vi "Smooth Ramp by Samples.vi"(8 "error in (no error)":errorcluster, 9 "End":dbl[](array[numeric]), 10 "Start":dbl[](array[numeric]), 11 "Generator in":refnum<class "Generator.lvclass">) -> (0 "Error out":errorcluster, 2 "Waveforms out":waveform(dbl)[](array[waveform]), 3 "Generator out":refnum<class "Generator.lvclass">)   [LabVIEW 2019, in "Generator.lvclass"]
uses:
  Generator.lvclass
  Generator.lvclass/Generator.ctl
  <vilib>/Analysis/NI_AALBase.lvlib
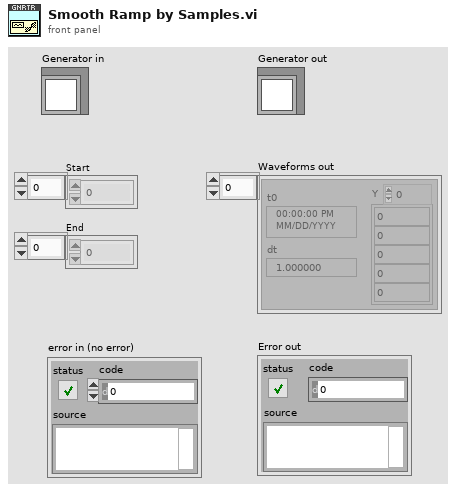
[diagram p1: front panel]
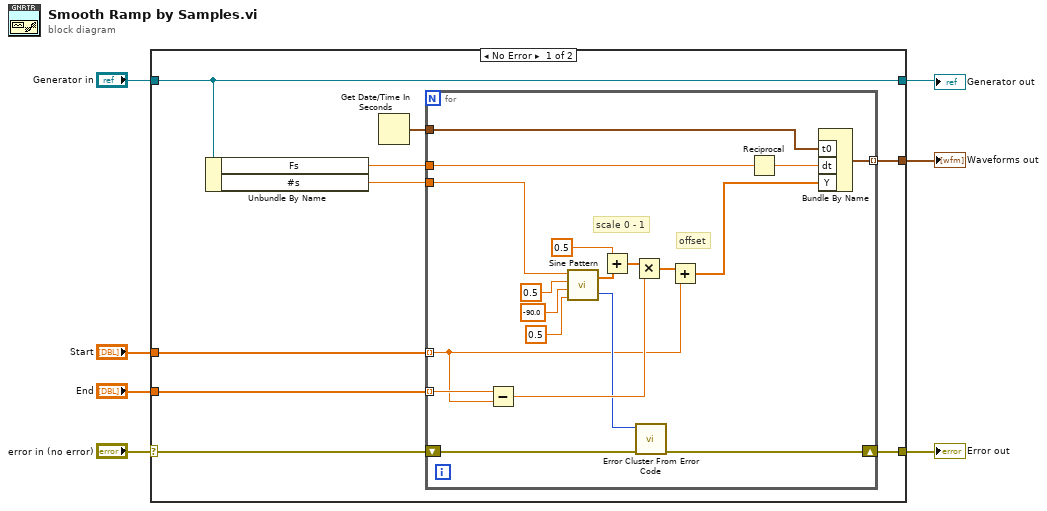
[diagram p0: block diagram]
diagram:
  n1 = case shown="No Error" "error in (no error)" {
    selector: "error in (no error)" -> [w14 w37]
    tunnel: "End" -> [w16 _]
    tunnel: [w15 w37] -> w5
    tunnel: [w12 _] -> w4
    tunnel: "Generator in" -> [w10 w36]
    tunnel: [w10 w36] -> w2
    tunnel: "Start" -> [w9 _]
    frame No Error {
      n2 = Unbundle By Name(w10) -> ("Fs"=w13:dbl, "#s"=w11:dbl)
      n3 = Get Date/Time In Seconds() -> (seconds since 1Jan1904=w8:timestamp)
      n4 = for {
        tunnel: w16 -> [w27] mode=indexing
        tunnel: w13 -> [w21]
        tunnel: [w20] -> w12 mode=indexing
        tunnel: w11 -> [w19]
        shift-right: [w25] -> w15
        shift-left: w14 -> [w24]
        tunnel: w9 -> [w18] mode=indexing
        tunnel: w8 -> [w17]
        # "offset"
        # "scale 0 - 1"
        n5 = Subtract(x=w27, y=w18) -> (x-y=w33:dbl)
        n6 = call <vilib>:"Sine Pattern.vi"("cycles"=0.5 ("cycles 2"), "phase(degrees)"=-90.0, "amplitude"=0.5, "samples"=w19) -> ("error"=w26:i32, "Sinusoidal Pattern"=w29:dbl[])
        n7 = Add(x=0.5 ("cycles 2"), y=w29) -> (x+y=w32:dbl[])
        n8 = Multiply(x=w32, y=w33) -> (x*y=w34:dbl[])
        n9 = call <vilib>:"Error Cluster From Error Code.vi"("error in (no error)"=w24, "error code (0)"=w26) -> ("error out"=w25:errorcluster)  [unwired: 7 in]
        n10 = Add(x=w34, y=w18) -> (x+y=w22:dbl[])
        n11 = Reciprocal(x=w21) -> (1/x=w23:dbl)
        n12 = Bundle By Name("t0"=w17, "dt"=w23, "Y"=w22) -> (w20:waveform(dbl))  [unwired: 1 in]
      }
    }
    frame Error {
    }
  }
  "Waveforms out" <- w4
  "Error out" <- w5
  "Generator out" <- w2
